vi "Copy State Name to Clipboard.vi"(11 "Tag":string) -> ()   [LabVIEW 2020]
uses:
  JKI State Machine API/source/JKI SM/JKI SM.lvclass
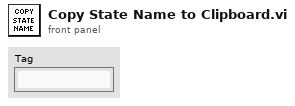
[diagram p1: front panel]
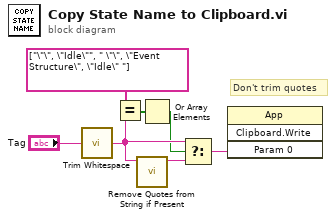
[diagram p0: block diagram]
diagram:
  # "Don't trim quotes"
  n1 = call <vilib>:"Trim Whitespace.vi"("string"="Tag") -> ("trimmed string"=w5:string)  [unwired: 1 in]
  n2 = Equal?(x=string[] ["\"\", \"Idle\"", " \"\", \"Event Structure\", \"Idle\" "], y=w5) -> (x = y?=w3:bool[])
  n3 = call "Remove Quotes from String if Present.vi"("String"=w5) -> ("String with Quotes Removed"=w6:string)  [unwired: 10 in]
  n4 = Or Array Elements(Boolean array=w3) -> (logical OR=w4:bool)
  n5 = Select(t=w5, s=w4, f=w6) -> (s? t:f=w7:string)
  n6 = invoke class="App" method="Clipboard.Write"("Param 0"=w7) -> ()  [unwired: 3 in, 4 out]
